vi "Create INI-Config.vi"(8 "error in":errorcluster, 11 "INI Filepath":path) -> (0 "error out":errorcluster, 3 "config-ini out":refnum<class "config-ini.lvclass">)   [LabVIEW 2020, in "hse-config.lvlib" / "config-ini.lvclass"]
doc: "Creates a new \"config-ini\" object based on the INI-file given.\n\n____\nHAMPEL SOFTWARE ENGINEERING v3.8.0 (2023-12-18 14:41)"
uses:
  config-ini.lvclass
  C:/GitLab-Runner/builds/7NHnU7RQc/0/open-source/hse-libraries/Source/hse-configuration/config-base/config-base.lvclass
  <vilib>/Utility/config.llb/Read Key (String).vi
  hse-misc/Conversion/ConvertStringToFloat_Scalar.vi
  config-ini.lvclass/config-ini.ctl
  <vilib>/Utility/config.llb/NI_LVConfig.lvlib
  hse-misc/hse-misc.lvlib
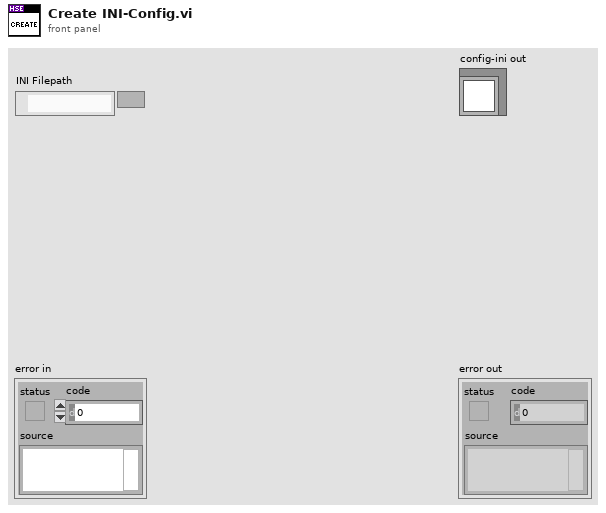
[diagram p1: front panel]
types:
  T1 = typedef "NI_LVConfig.lvlib/Config Data RefNum.ctl" = refnum<k1>
  T2 = typedef "NI_Data Type.lvlib/Data Type.ctl" = enum8{"Invalid Type", "Void", "I8", "I16", "I32", "I64", "U8", "U16", "U32", "U64", "Single Float", "Double Float", "Extended Float", "Single Complex", "Double Complex", "Extended Complex", "Enum U8", "Enum U16", "Enum U32", "Enum U64", "Single Float With Unit", "Double Float With Unit", "Extended Float With Unit", "Single Complex with Unit", "Double Complex with Unit", "Extended Complex with Unit", "Boolean", "String", "Path", "Picture", "Tag", "Array", "Cluster", "Variant", "LV Variant", "Waveform", "Timestamp", "Digital Waveform", "Digital Data", "ExpressData", "Refnum", "External Data", "VI", "Poly VI", "LabVIEW Class Instance", "Fixed Point", "Set Collection", "Map Collection"}
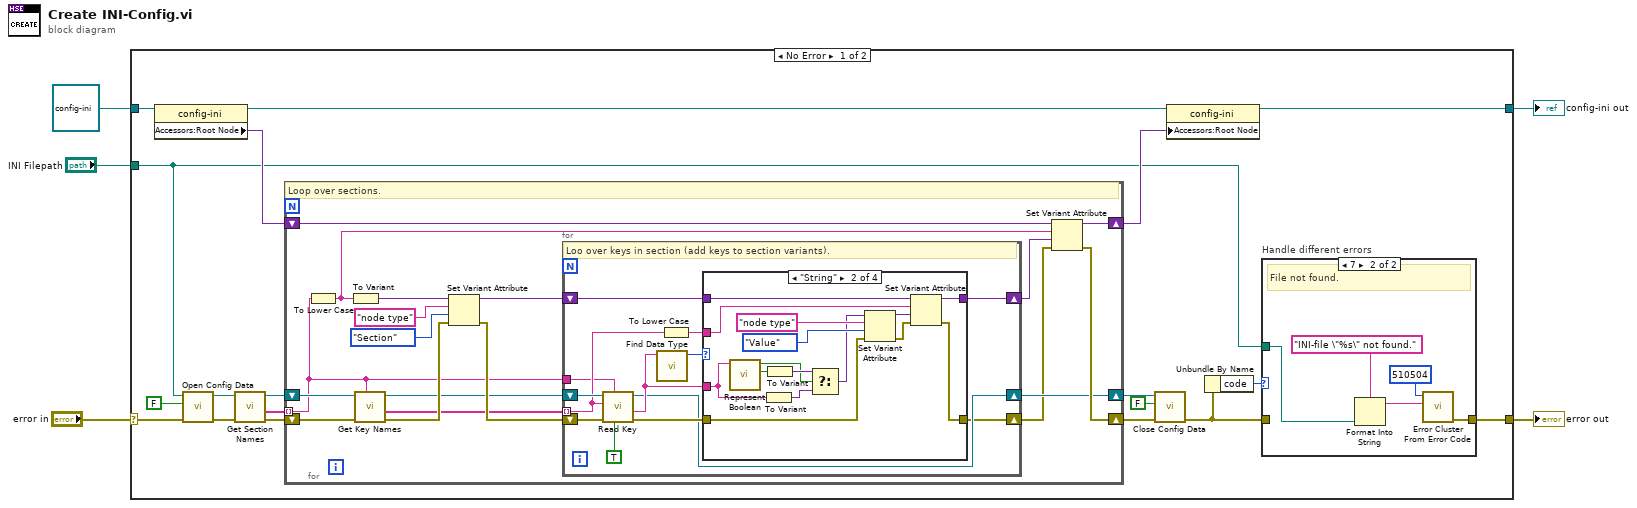
[diagram p0: block diagram]
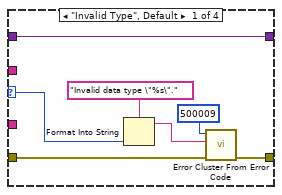
[diagram p3: hidden frame]
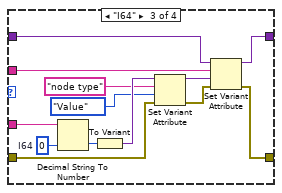
[diagram p4: hidden frame]
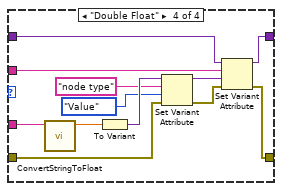
[diagram p5: hidden frame]
diagram:
  n1 = case shown="No Error" "error in" {
    selector: "error in" -> [w23 w110]
    tunnel: [w7 w110] -> w4
    tunnel: [w12 w109] -> w2
    tunnel: refnum<class "config-ini.lvclass"> refnum ("config-ini in") -> [w24 w109]
    tunnel: "INI Filepath" -> [w6 _]
    frame No Error {
      n2 = property class="config-ini"(reference=w24) -> (reference out=w16:refnum<class "config-ini.lvclass">, "Accessors:Root Node"=w15:variant)  [unwired: 1 in, 1 out]
      n3 = call <vilib>:"Open Config Data.vi"("error in (no error)"=w23, "create file if necessary (T)"=FALSE, "configuration file path"=w6) -> ("error out"=w21:errorcluster, "refnum"=w20:T1)  [unwired: 6 in, 1 out]
      n4 = call <vilib>:"Get Section Names.vi"("error in (no error)"=w21, "refnum"=w20) -> ("error out"=w19:errorcluster, "section names"=w17:string[], "refnum out"=w18:T1)  [unwired: 7 in]
      n5 = for {
        tunnel: w17 -> [w33] mode=indexing
        shift-right: [w34] -> w11
        shift-left: w15 -> [w35]
        shift-right: [w48] -> w13
        shift-left: w19 -> [w45]
        shift-right: [w38] -> w14
        shift-left: w18 -> [w44]
        # "Loop over sections."
        n6 = To Lower Case(string=w33) -> (all lower case string=w31:string)
        n7 = To Variant(anything=w31) -> (Variant=w40:variant)
        n8 = call <vilib>:"Get Key Names.vi"("section"=w33, "error in (no error)"=w45, "refnum"=w44) -> ("error out"=w46:errorcluster, "key names"=w42:string[], "refnum out"=w43:T1)  [unwired: 5 in, 1 out]
        n9 = Set Variant Attribute(Variant=w40, name="node type", value=enum8{"Root", "Section", "Value"}."Section" ("Node Type"), error in=w46) -> (Variant out=w39:variant, error out=w47:errorcluster)  [unwired: 1 out]
        n10 = for {
          tunnel: w42 -> [w55] mode=indexing
          tunnel: w33 -> [w53]
          shift-right: [w52] -> w32
          shift-left: w47 -> [w61]
          shift-right: [w51] -> w36
          shift-left: w39 -> [w56]
          shift-right: [w54] -> w38
          shift-left: w43 -> [w60]
          # "Loo over keys in section (add keys to section variants)."
          n11 = call-poly <vilib>:"Read Key.vi"("read raw string? (F)"=TRUE, "section"=w53, "error in (no error)"=w61, "key"=w55, "refnum"=w60) -> ("error out"=w57:errorcluster, "value"=w58:string, "refnum out"=w54:T1)  [unwired: 3 in, 1 out]
          n12 = call "Find Data Type.vi"("String"=w58) -> ("Data Type"=w59:T2)  [unwired: 10 in]
          n13 = To Lower Case(string=w55) -> (all lower case string=w50:string)
          n14 = case shown="\"String\"" w59 {
            selector: w59 -> [w62 _ _ _]
            tunnel: w58 -> [_ w75 w96 w101]
            tunnel: w57 -> [w67 w79 w92 w107]
            tunnel: w56 -> [w68 w81 w91 w106]
            tunnel: w50 -> [_ w69 w84 w97]
            tunnel: [w68 w80 w90 w103] -> w51
            tunnel: [w63 w78 w89 w102] -> w52
            frame "Invalid Type", Default {
              n15 = Format Into String(format string="Invalid data type \"%s\".", w62) -> (resulting string=w65:string)  [unwired: 2 in, 1 out]
              n16 = call <vilib>:"Error Cluster From Error Code.vi"("error in (no error)"=w67, "error message (\"\")"=w65, "error code (0)"=500009) -> ("error out"=w63:errorcluster)  [unwired: 6 in]
            }
            frame "String" {
              n17 = call "Represent Boolean.vi"("String"=w75) -> ("Value"=w74:bool, "Represent Boolean?"=w72:bool)  [unwired: 9 in]
              n18 = To Variant(anything=w75) -> (Variant=w70:variant)
              n19 = To Variant(anything=w74) -> (Variant=w73:variant)
              n20 = Select(t=w73, s=w72, f=w70) -> (s? t:f=w71:variant)
              n21 = Set Variant Attribute(Variant=w71, name="node type", value=enum8{"Root", "Section", "Value"}."Value" ("Node Type"), error in=w79) -> (Variant out=w83:variant, error out=w82:errorcluster)  [unwired: 1 out]
              n22 = Set Variant Attribute(Variant=w81, name=w69, value=w83, error in=w82) -> (Variant out=w80:variant, error out=w78:errorcluster)  [unwired: 1 out]
            }
            frame "I64" {
              w95 = i64 0  # I64
              n23 = Decimal String To Number(string=w96, default (0L)=w95) -> (number=w94:i64)  [unwired: 1 in, 1 out]
              n24 = To Variant(anything=w94) -> (Variant=w93:variant)
              n25 = Set Variant Attribute(Variant=w93, name="node type", value=enum8{"Root", "Section", "Value"}."Value" ("Node Type"), error in=w92) -> (Variant out=w88:variant, error out=w87:errorcluster)  [unwired: 1 out]
              n26 = Set Variant Attribute(Variant=w91, name=w84, value=w88, error in=w87) -> (Variant out=w90:variant, error out=w89:errorcluster)  [unwired: 1 out]
            }
            frame "Double Float" {
              n27 = call-poly "ConvertStringToFloat.vi"("String"=w101) -> ("Double"=w100:dbl)  [unwired: 9 in, 1 out]
              n28 = To Variant(anything=w100) -> (Variant=w108:variant)
              n29 = Set Variant Attribute(Variant=w108, name="node type", value=enum8{"Root", "Section", "Value"}."Value" ("Node Type"), error in=w107) -> (Variant out=w105:variant, error out=w104:errorcluster)  [unwired: 1 out]
              n30 = Set Variant Attribute(Variant=w106, name=w97, value=w105, error in=w104) -> (Variant out=w103:variant, error out=w102:errorcluster)  [unwired: 1 out]
            }
          }
        }
        n31 = Set Variant Attribute(Variant=w35, name=w31, value=w36, error in=w32) -> (Variant out=w34:variant, error out=w48:errorcluster)  [unwired: 1 out]
      }
      n32 = call <vilib>:"Close Config Data.vi"("error in (no error)"=w13, "write file if changed (T)"=FALSE, "refnum"=w14) -> ("error out"=w9:errorcluster)  [unwired: 7 in, 1 out]
      n33 = property class="config-ini"(reference=w16, "Accessors:Root Node"=w11) -> (reference out=w12:refnum<class "config-ini.lvclass">)  [unwired: 1 in, 1 out]
      n34 = Unbundle By Name(w9) -> ("code"=w8:i32)
      n35 = case "Handle different errors" shown="7" w8 {
        tunnel: w9 -> [w25 _]
        tunnel: [w25 w30] -> w7
        tunnel: w6 -> [_ w26]
        frame 0, Default {
          # "No error and all not handled errors."
        }
        frame 7 {
          # "File not found."
          n36 = Format Into String(format string="INI-file \"%s\" not found.", w26) -> (resulting string=w28:string)  [unwired: 2 in, 1 out]
          n37 = call <vilib>:"Error Cluster From Error Code.vi"("error message (\"\")"=w28, "error code (0)"=510504) -> ("error out"=w30:errorcluster)  [unwired: 7 in]
        }
      }
    }
    frame Error {
    }
  }
  "error out" <- w4
  "config-ini out" <- w2
